vi "Get message from save image VI.vi"(8 "error in (no error)":errorcluster, 11 "Channel in":refnum<class "Channel.lvclass">) -> (0 "error out":errorcluster, 3 "Channel out":refnum<class "Channel.lvclass">)   [LabVIEW 2018, in "Channel.lvclass"]
doc: "Get message from the save image VI"
uses:
  Channel.lvclass
  Channel.lvclass/Channel.ctl
  RxTx/CCS_RxTx.lvclass
  Simulated_CCD_Camera/Simulated Camera.lvclass
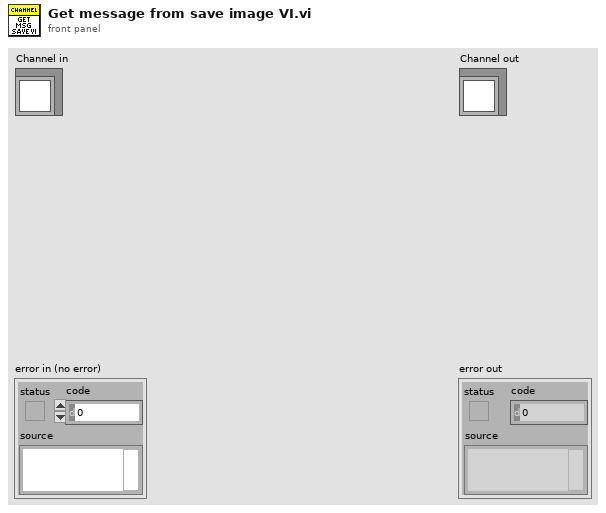
[diagram p1: front panel]
types:
  T1 = cluster{"CYCLES_DONE":u16, "LAST_IMAGE_NAME":string, "USED_DISK_SPACE":u16, "FRAMES_DONE":u16, "CCD_STATUS":string, "CURRENT_TEMPERATURE":i16, "TEMPERATURE_STATUS":string, "FRAME_EXPOSURE_TIME":sgl, "ERROR":bool, "SERIAL_NUMBER":u16, "ACQUIRING":bool, "IMAGE_INDEX":u32, "SEQS_DONE":u16}
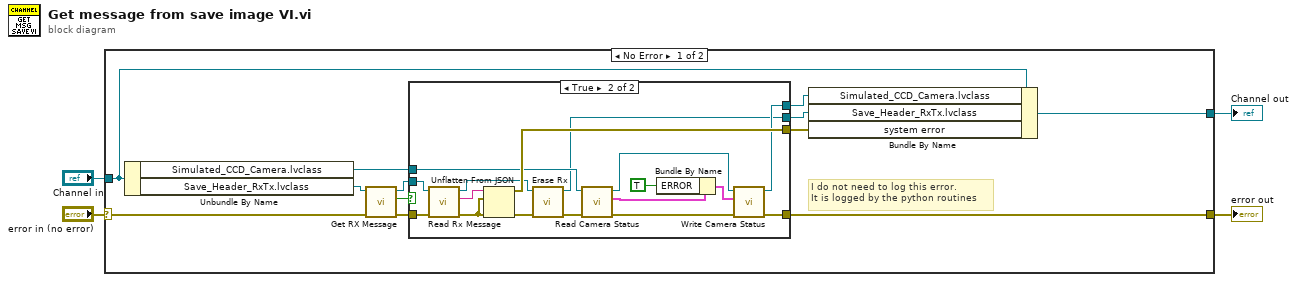
[diagram p0: block diagram]
diagram:
  n1 = case shown="No Error" "error in (no error)" {
    selector: "error in (no error)" -> [w14 w38]
    tunnel: [w10 w38] -> w3
    tunnel: [w9 w37] -> w1
    tunnel: "Channel in" -> [w16 w37]
    frame No Error {
      # "I do not need to log this error.\nIt is logged by the python routines"
      n2 = Unbundle By Name(w16) -> ("Simulated_CCD_Camera.lvclass"=w5:refnum<class "Simulated Camera.lvclass">, "Save_Header_RxTx.lvclass"=w15:refnum<class "CCS_RxTx.lvclass">)
      n3 = call "Get RX Message.vi"("error in (no error)"=w14, "RxTx in"=w15) -> ("error out"=w13:errorcluster, "new msg"=w8:bool, "RxTx out"=w12:refnum<class "CCS_RxTx.lvclass">)  [unwired: 7 in]
      n4 = case shown="True" w8 {
        tunnel: w13 -> [w18 w34]
        tunnel: w12 -> [w19 w35]
        tunnel: [w19 w21] -> w11
        tunnel: [w18 w24] -> w10
        tunnel: [_ w36] -> w7
        tunnel: [w17 w23] -> w6
        tunnel: w5 -> [w17 w22]
        frame False {
        }
        frame True {
          n5 = call "Read Rx Message.vi"("error in (no error)"=w34, "RxTx in"=w35) -> ("error out"=w32:errorcluster, "Rx Message"=w33:string, "RxTx out"=w31:refnum<class "CCS_RxTx.lvclass">)  [unwired: 7 in]
          n6 = Unflatten From JSON(JSON string=w33, type and defaults=w32, error in (no error)=w32) -> (value=w36:errorcluster, error out=w30:errorcluster)  [unwired: 4 in]
          n7 = call "Erase Rx.vi"("error in (no error)"=w30, "RxTx in"=w31) -> ("error out"=w25:errorcluster, "RxTx out"=w21:refnum<class "CCS_RxTx.lvclass">)  [unwired: 8 in]
          n8 = call "Read Camera Status.vi"("error in (no error)"=w25, "CCDCamera in"=w22) -> ("error out"=w29:errorcluster, "Camera Status"=w28:T1, "CCDCamera out"=w20:refnum<class "Simulated Camera.lvclass">)  [unwired: 7 in]
          n9 = Bundle By Name(cluster=w28, "ERROR"=TRUE) -> (w27:T1)
          n10 = call "Write Camera Status.vi"("error in (no error)"=w29, "Camera Status"=w27, "CCDCamera in"=w20) -> ("error out"=w24:errorcluster, "CCDCamera out"=w23:refnum<class "Simulated Camera.lvclass">)  [unwired: 7 in]
        }
      }
      n11 = Bundle By Name(cluster=w16, "Simulated_CCD_Camera.lvclass"=w6, "Save_Header_RxTx.lvclass"=w11, "system error"=w7) -> (w9:refnum<class "Channel.lvclass">)
    }
    frame Error {
    }
  }
  "error out" <- w3
  "Channel out" <- w1
